vi "Draw Bone.vi"(4 "Body Index":i32, 6 "Color":u32(colorbox)=16711680, 7 "Include Inferred Joints?":bool=TRUE, 8 "error in":errorcluster, 9 "Ending Joint":T1=2 items=["SpineBase", "SpineMid", "Neck", "Head", "ShoulderLeft", "ElbowLeft", "WristLeft", "HandLeft", "ShoulderRight", "ElbowRight", "WristRight", "HandRight", "HipLeft", "KneeLeft", "AnkleLeft", "FootLeft", "HipRight", "KneeRight", "AnkleRight", "FootRight", "SpineShoulder", "HandTipLeft", "ThumbLeft", "HandTipRight", "ThumbRight"], 10 "Starting Joint":T1=3 items=["SpineBase", "SpineMid", "Neck", "Head", "ShoulderLeft", "ElbowLeft", "WristLeft", "HandLeft", "ShoulderRight", "ElbowRight", "WristRight", "HandRight", "HipLeft", "KneeLeft", "AnkleLeft", "FootLeft", "HipRight", "KneeRight", "AnkleRight", "FootRight", "SpineShoulder", "HandTipLeft", "ThumbLeft", "HandTipRight", "ThumbRight"], 11 "Image":T2) -> (0 "error out":errorcluster, 3 "Image Out":T2)   [LabVIEW 2014, in "LVH-KinectOne.lvlib"]
uses:
  LVH-KinectOne.lvlib
  <vilib>/vision/Image Controls.llb/IMAQ Image.ctl
  Type Defs/JointType.ctl
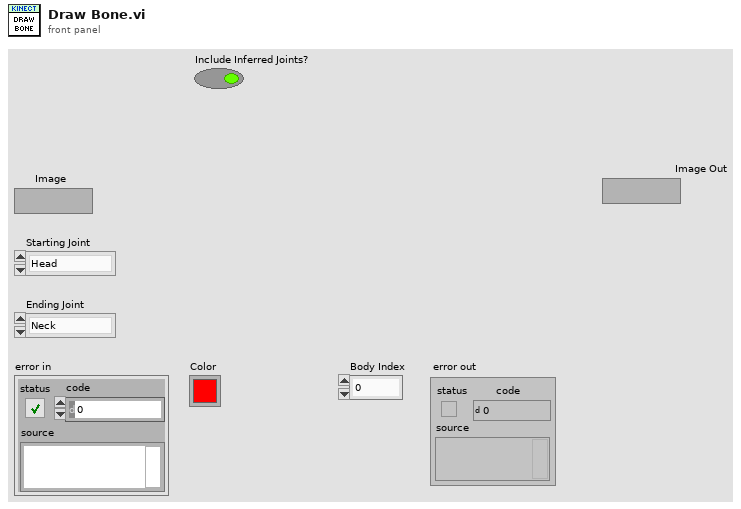
[diagram p1: front panel]
types:
  T1 = typedef "LVH-KinectOne.lvlib/JointType.ctl" = i32
  T2 = typedef "IMAQ Image.ctl" = refnum<image>
  T3 = typedef "LVH-KinectOne.lvlib/Joint Position.ctl" = cluster{"Position":cluster{"X":sgl, "Y":sgl}, "TrackingState":i32}
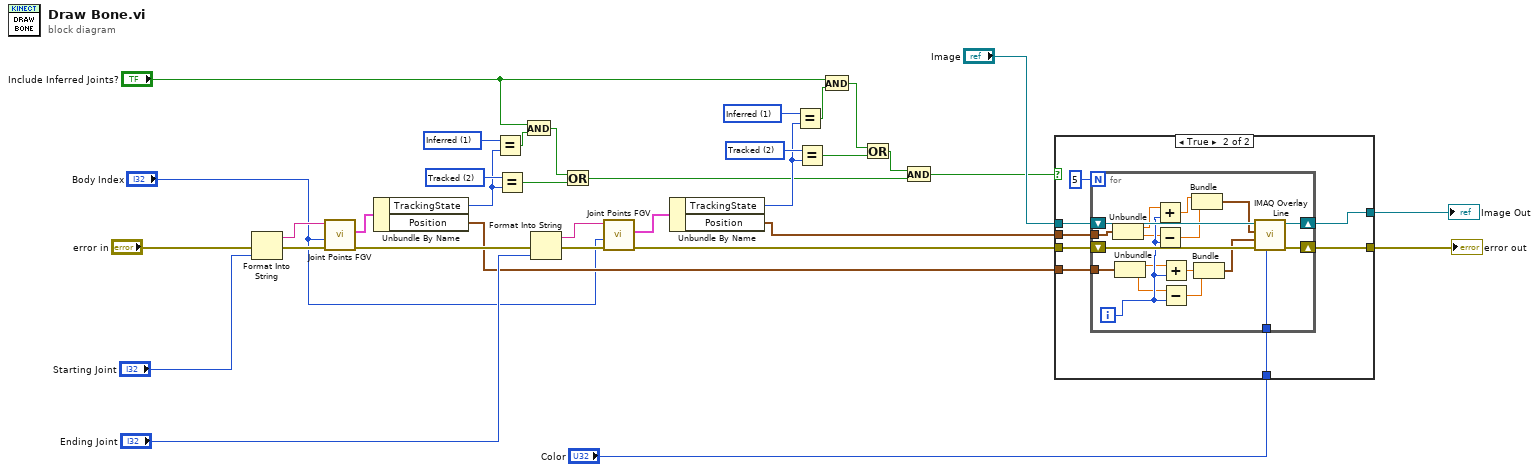
[diagram p0: block diagram]
diagram:
  w11 = 2 items=["NotTracked", "Inferred", "Tracked"] ("TrackingState")
  w10 = 1 items=["NotTracked", "Inferred", "Tracked"] ("TrackingState")
  w19 = 2 items=["NotTracked", "Inferred", "Tracked"] ("TrackingState")
  w20 = 1 items=["NotTracked", "Inferred", "Tracked"] ("TrackingState")
  n1 = Format Into String(error in="error in", "Starting Joint") -> (resulting string=w22:string, error out=w28:errorcluster)  [unwired: 2 in]
  n2 = call "Joint Points FGV.vi"("error in (no error)"=w28, "Body Index"="Body Index", "name"=w22) -> ("error out"=w26:errorcluster, "Joint Position"=w21:T3)  [unwired: 7 in]
  n3 = Unbundle By Name(w21) -> ("TrackingState"=w18:i32, "Position"=w2:cluster{"X":sgl, "Y":sgl})
  n4 = Equal?(x=w20, y=w18) -> (x = y?=w17:bool)
  n5 = Equal?(x=w19, y=w18) -> (x = y?=w15:bool)
  n6 = And(x="Include Inferred Joints?", y=w17) -> (x .and. y?=w16:bool)
  n7 = Format Into String(error in=w26, "Ending Joint") -> (resulting string=w25:string, error out=w27:errorcluster)  [unwired: 2 in]
  n8 = Or(x=w16, y=w15) -> (x .or. y?=w6:bool)
  n9 = call "Joint Points FGV.vi"("error in (no error)"=w27, "Body Index"="Body Index", "name"=w25) -> ("error out"=w24:errorcluster, "Joint Position"=w23:T3)  [unwired: 7 in]
  n10 = Unbundle By Name(w23) -> ("TrackingState"=w9:i32, "Position"=w3:cluster{"X":sgl, "Y":sgl})
  n11 = Equal?(x=w10, y=w9) -> (x = y?=w12:bool)
  n12 = Equal?(x=w11, y=w9) -> (x = y?=w14:bool)
  n13 = And(x="Include Inferred Joints?", y=w12) -> (x .and. y?=w13:bool)
  n14 = Or(x=w13, y=w14) -> (x .or. y?=w7:bool)
  n15 = And(x=w7, y=w6) -> (x .and. y?=w5:bool)
  n16 = case shown="True" w5 {
    tunnel: "Image" -> [w35 w44]
    tunnel: [w36 w43] -> w33
    tunnel: [w35 w42] -> w32
    tunnel: "Color" -> [_ w41]
    tunnel: w24 -> [w36 w40]
    tunnel: w3 -> [_ w38]
    tunnel: w2 -> [_ w37]
    frame False {
    }
    frame True {
      n17 = for {
        N: 5 -> [_]
        shift-right: [w60] -> w43
        shift-left: w40 -> [w62]
        shift-right: [w59] -> w42
        shift-left: w44 -> [w61]
        tunnel: w41 -> [w51]
        tunnel: w38 -> [w50]
        tunnel: w37 -> [w49]
        i -> [w58]
        n18 = Unbundle(w50) -> ("X"=w48:sgl, "Y"=w47:sgl)
        n19 = Unbundle(w49) -> ("X"=w46:sgl, "Y"=w45:sgl)
        n20 = Add(x=w48, y=w58) -> (x+y=w57:sgl)
        n21 = Subtract(x=w47, y=w58) -> (x-y=w56:sgl)
        n22 = Add(x=w46, y=w58) -> (x+y=w54:sgl)
        n23 = Subtract(x=w45, y=w58) -> (x-y=w53:sgl)
        n24 = Bundle(w57, w56) -> (w55:cluster{sgl, sgl})  [unwired: 1 in]
        n25 = Bundle(w54, w53) -> (w52:cluster{sgl, sgl})  [unwired: 1 in]
        n26 = call "IMAQ Overlay Line"("Color"=w51, "error in (no error)"=w62, "End Point"=w52, "Start Point"=w55, "Image"=w61) -> ("error out"=w60:errorcluster, "Image Out"=w59:T2)  [unwired: 5 in]
      }
    }
  }
  "error out" <- w33
  "Image Out" <- w32
